vi "Zero Lift.vi"() -> (2 "Boolean":bool)   [LabVIEW 2014]
uses:
  <vilib>/Rock Robotics/WPI/SafetyOutput/WPI_SafetyOutputConfigMenu.ctl
  Robot Global Data.vi
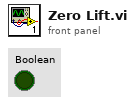
[diagram p1: front panel]
types:
  T1 = typedef "WPI_SafetyOutputConfigMenu.ctl" = enum16{"Enable", "Disable"}
  T2 = typedef "WPI_MotorControlDeviceRef.ctl" = cluster{"DeviceStatus":errorcluster, "Type":T3, "PWM":cluster{"Controller":T4, "PWM Channel":T5, "DeadBand":T6}, "CAN":cluster{"Device Number":u8, "Control Mode":T7, "Semaphore":T8, "Max Vout":dbl, "TalonSRX Control Mode":T9}, "Invert":bool, "TransformRef":T10, "InvTransformRef":T10}
  T3 = typedef "WPI_MotorControlType.ctl" = enum16{"PWM", "CAN", "CANTalonSRX"}
  T4 = typedef "FPGA_TypedefDigitalModule.ctl" = enum16{"Controller 1"}
  T5 = typedef "FPGA_DIOPWMChannel.ctl" = enum8{"PWM 0", "PWM 1", "PWM 2", "PWM 3", "PWM 4", "PWM 5", "PWM 6", "PWM 7", "PWM 8", "PWM 9", "PWM MXP 0", "PWM MXP 1", "PWM MXP 2", "PWM MXP 3", "PWM MXP 4", "PWM MXP 5", "PWM MXP 6", "PWM MXP 7", "PWM MXP 8", "PWM MXP 9", "Invalid"}
  T6 = typedef "WPI_PWMDeadband.ctl" = cluster{"Name":string, "maxPositivePwm":i32, "minPositivePwm":i32, "centerPwm":i32, "maxNegativePwm":i32, "minNegativePwm":i32, "angularRange":u16}
  T7 = typedef "WPI_CANJaguar_ControlMode.ctl" = enum8{"Percent VBus", "Current", "Speed", "Position", "Voltage"}
  T8 = typedef "Semaphore RefNum" = refnum<k1>
  T9 = typedef "WPI_CANTalonSRX_APIControlMode.ctl" = enum8{"Percent VBus", "Speed", "Position", "Slave", "Unchanged / Invalid"}
  T10 = typedef "WPI_PWMTransform_ConPane.ctl" = refnum<vi>
  T11 = typedef "WPI_EncoderDevRef.ctl" = cluster{"DevStatus":errorcluster, "EncoderIndex":T12, "CounterIndex":T13, "DistancePerCount":dbl, "Decoding Type":T14}
  T12 = typedef "FPGA_EncoderIdx.ctl" = enum8{"Enc 0", "Enc 1", "Enc 2", "Enc 3", "Enc 4", "Enc 5", "Enc 6", "Enc 7", "Invalid"}
  T13 = typedef "FPGA_CounterCtrSystemIndex.ctl" = enum8{"Ctr 0", "Ctr 1", "Ctr 2", "Ctr 3", "Ctr 4", "Ctr 5", "Ctr 6", "Ctr 7", "Invalid"}
  T14 = typedef "WPI_EncoderType.ctl" = enum16{"1x", "2x", "4x"}
  T15 = typedef "WPI_DigitalInputDevRef.ctl" = cluster{"DevStatus":errorcluster, "DIO Channel":T16, "Controller":T4}
  T16 = typedef "FPGA_DIOChannel.ctl" = enum8{"DIO 0", "DIO 1", "DIO 2", "DIO 3", "DIO 4", "DIO 5", "DIO 6", "DIO 7", "DIO 8", "DIO 9", "DIO MXP 0", "DIO MXP 1", "DIO MXP 2", "DIO MXP 3", "DIO MXP 4", "DIO MXP 5", "DIO MXP 6", "DIO MXP 7", "DIO MXP 8", "DIO MXP 9", "DIO MXP 10", "DIO MXP 11", "DIO MXP 12", "DIO MXP 13", "DIO MXP 14", "DIO MXP 15", "Invalid"}
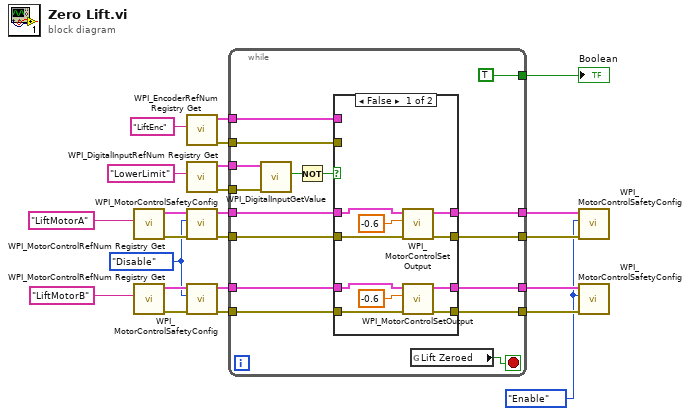
[diagram p0: block diagram]
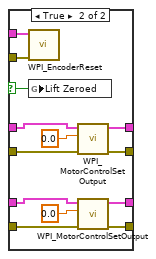
[diagram p2: hidden frame]
diagram:
  w2 = WPI_SafetyOutputConfigMenu."Enable" ("mode")
  w1 = WPI_SafetyOutputConfigMenu."Disable" ("mode")
  n1 = call <vilib>:"WPI_MotorControlRefNum Registry Get.vi"("refnum name"="LiftMotorA") -> ("error out"=w8:errorcluster, "MotorControlDevRef"=w7:T2)  [unwired: 9 in]
  n2 = call <vilib>:"WPI_MotorControlRefNum Registry Get.vi"("refnum name"="LiftMotorB") -> ("error out"=w15:errorcluster, "MotorControlDevRef"=w14:T2)  [unwired: 9 in]
  n3 = call <vilib>:"WPI_EncoderRefNum Registry Get.vi"("refnum name"="LiftEnc") -> ("error out"=w16:errorcluster, "EncoderDevRef"=w17:T11)  [unwired: 9 in]
  n4 = call <vilib>:"WPI_DigitalInputRefNum Registry Get.vi"("refnum name"="LowerLimit") -> ("error out"=w20:errorcluster, "DigitalInputDevRef"=w21:T15)  [unwired: 9 in]
  n5 = call <vilib>:"WPI_MotorControlSafetyConfig.vi"("error in (no error)"=w8, "mode"=w1, "MotorControlDevRef"=w7) -> ("error out"=w5:errorcluster, "MotorControlDevRef"=w6:T2)  [unwired: 7 in]
  n6 = call <vilib>:"WPI_MotorControlSafetyConfig.vi"("error in (no error)"=w15, "mode"=w1, "MotorControlDevRef"=w14) -> ("error out"=w12:errorcluster, "MotorControlDevRef"=w13:T2)  [unwired: 7 in]
  n7 = while {
    tunnel: w21 -> [w36]
    tunnel: w20 -> [w35]
    tunnel: w13 -> [w34]
    tunnel: w12 -> [w33]
    tunnel: [TRUE] -> w19
    tunnel: w17 -> [w31]
    tunnel: w16 -> [w30]
    tunnel: [w29] -> w11
    tunnel: [w28] -> w10
    tunnel: w6 -> [w27]
    tunnel: w5 -> [w26]
    tunnel: [w25] -> w4
    tunnel: [w24] -> w3
    stop <- w39 stop-if-true
    n8 = call <vilib>:"WPI_DigitalInputGetValue.vi"("error in (no error)"=w35, "DigitalInputDevRef"=w36) -> ("Value"=w38:bool)  [unwired: 7 in, 2 out]
    n9 = Not(x=w38) -> (.not. x?=w37:bool)
    n10 = case shown="False" w37 {
      selector: w37 -> [_ w59]
      tunnel: w34 -> [w48 w61]
      tunnel: w33 -> [w47 w60]
      tunnel: w31 -> [_ w58]
      tunnel: w30 -> [_ w57]
      tunnel: [w46 w56] -> w29
      tunnel: [w45 w55] -> w28
      tunnel: w27 -> [w41 w53]
      tunnel: w26 -> [w40 w52]
      tunnel: [w42 w51] -> w25
      tunnel: [w43 w50] -> w24
      frame False {
        n11 = call <vilib>:"WPI_MotorControlSetOutput.vi"("error in (no error)"=w40, "Output"=-0.6, "MotorControlDevRef"=w41) -> ("error out"=w42:errorcluster, "MotorControlDevRef"=w43:T2)  [unwired: 6 in, 1 out]
        n12 = call <vilib>:"WPI_MotorControlSetOutput.vi"("error in (no error)"=w47, "Output"=-0.6, "MotorControlDevRef"=w48) -> ("error out"=w45:errorcluster, "MotorControlDevRef"=w46:T2)  [unwired: 6 in, 1 out]
      }
      frame True {
        n13 = call <vilib>:"WPI_EncoderReset.vi"("error in (no error)"=w57, "EncoderDevRef"=w58) -> ()  [unwired: 8 in, 2 out]
        n14 = global write "Robot Global Data.vi" "Lift Zeroed"(w59) -> ()
        n15 = call <vilib>:"WPI_MotorControlSetOutput.vi"("error in (no error)"=w52, "Output"=0.0, "MotorControlDevRef"=w53) -> ("error out"=w51:errorcluster, "MotorControlDevRef"=w50:T2)  [unwired: 6 in, 1 out]
        n16 = call <vilib>:"WPI_MotorControlSetOutput.vi"("error in (no error)"=w60, "Output"=0.0, "MotorControlDevRef"=w61) -> ("error out"=w55:errorcluster, "MotorControlDevRef"=w56:T2)  [unwired: 6 in, 1 out]
      }
    }
    n17 = global read "Robot Global Data.vi" "Lift Zeroed"() -> (w39:bool)
  }
  "Boolean" <- w19
  n18 = call <vilib>:"WPI_MotorControlSafetyConfig.vi"("error in (no error)"=w4, "mode"=w2, "MotorControlDevRef"=w3) -> ()  [unwired: 7 in, 2 out]
  n19 = call <vilib>:"WPI_MotorControlSafetyConfig.vi"("error in (no error)"=w10, "mode"=w2, "MotorControlDevRef"=w11) -> ()  [unwired: 7 in, 2 out]
